vi "Global_Init.vi"(11 "Object":T1) -> ()   [LabVIEW 2020, in "FlexWorker_Provider.lvlib"]
uses:
  FlexWorker_Provider.lvlib
  <resource>/Framework/Providers/API/mxLvOverlayAlias.ctl
  <resource>/Framework/Providers/API/ItemRef.ctl
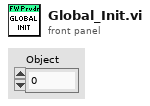
[diagram p1: front panel]
types:
  T1 = typedef "ItemRef.ctl" = u64
  T2 = typedef "mxLvOverlayAlias.ctl" = cluster{"Overlay Alias":string, "Icon File Name":path}
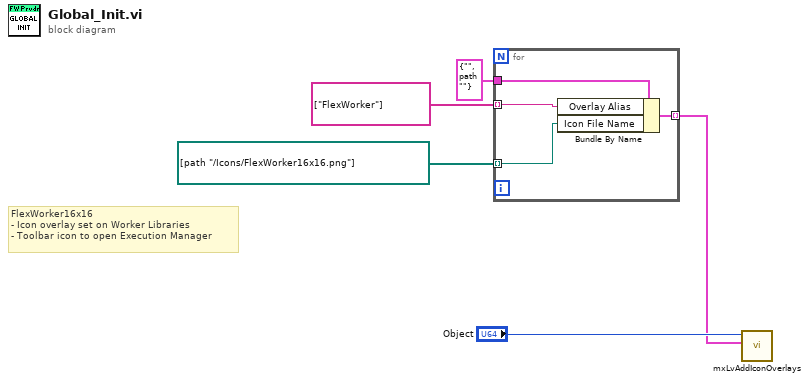
[diagram p0: block diagram]
diagram:
  # "FlexWorker16x16\n- Icon overlay set on Worker Libraries\n- Toolbar icon to open Execution Manager"
  n1 = for {
    tunnel: T2 {"Overlay Alias"="", "Icon File Name"=path ""} ("Icon Overlay Alias") -> [w9]
    tunnel: [w8] -> w1 mode=indexing
    tunnel: string[] ["FlexWorker"] ("overlay alias") -> [w7] mode=indexing
    tunnel: path[] [path "../Icons/FlexWorker16x16.png"] ("icon filename") -> [w6] mode=indexing
    n2 = Bundle By Name(cluster=w9, "Overlay Alias"=w7, "Icon File Name"=w6) -> (w8:T2)
  }
  n3 = call <resource>:"mxLvAddIconOverlays.vi"("Overlay Aliases"=w1, "Item"="Object") -> ()  [unwired: 8 in, 2 out]
